vi "Read Results.vi"(8 "error in":errorcluster, 11 "Results Directory":path) -> (0 "error out":errorcluster, 3 "Results":T1[](array[typedef]))   [LabVIEW 2020, in "Peer Review.lvclass"]
uses:
  Peer Review.lvclass
  TypeDefs/File Info.ctl
  TypeDefs/File State.ctl
  TypeDefs/VI Type.ctl
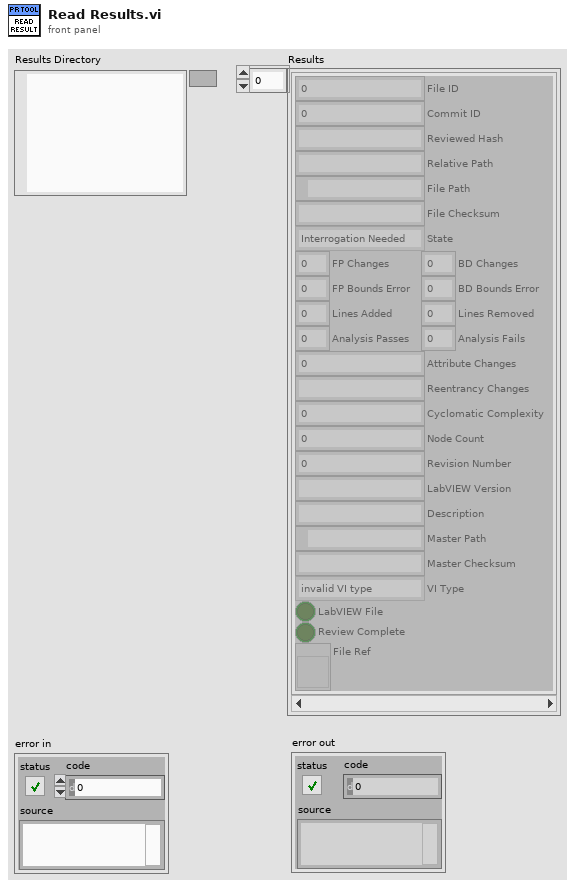
[diagram p1: front panel]
types:
  T1 = typedef "Peer Review.lvclass/File Info.ctl" = cluster{"File ID":i32, "Commit ID":i32, "Reviewed Hash":string, "Relative Path":string, "File Path":path, "File Checksum":string, "State":T2, "FP Changes":i32, "BD Changes":i32, "FP Bounds Error":dbl, "BD Bounds Error":dbl, "Lines Added":i32, "Lines Removed":i32, "Analysis Passes":i32, "Analysis Fails":i32, "Attribute Changes":i32, "Reentrancy Changes":string, "Cyclomatic Complexity":i32, "Node Count":i32, "Revision Number":u32, "LabVIEW Version":string, "Description":string, "Master Path":path, "Master Checksum":string, "VI Type":T3, "LabVIEW File":bool, "Review Complete":bool, "File Ref":refnum<vi>}
  T2 = typedef "Peer Review.lvclass/File State.ctl" = enum16{"Interrogation Needed", "Modified", "Deleted", "Added", "Matches Previous", "No Changes", "Moved"}
  T3 = typedef "Peer Review.lvclass/VI Type.ctl" = enum32{"invalid VI type", "Standard VI", "Control VI", "Global VI", "Polymorphic VI", "Configuration VI", "SubSystem", "Facade VI", "Method VI", "Statechart Diagram VI"}
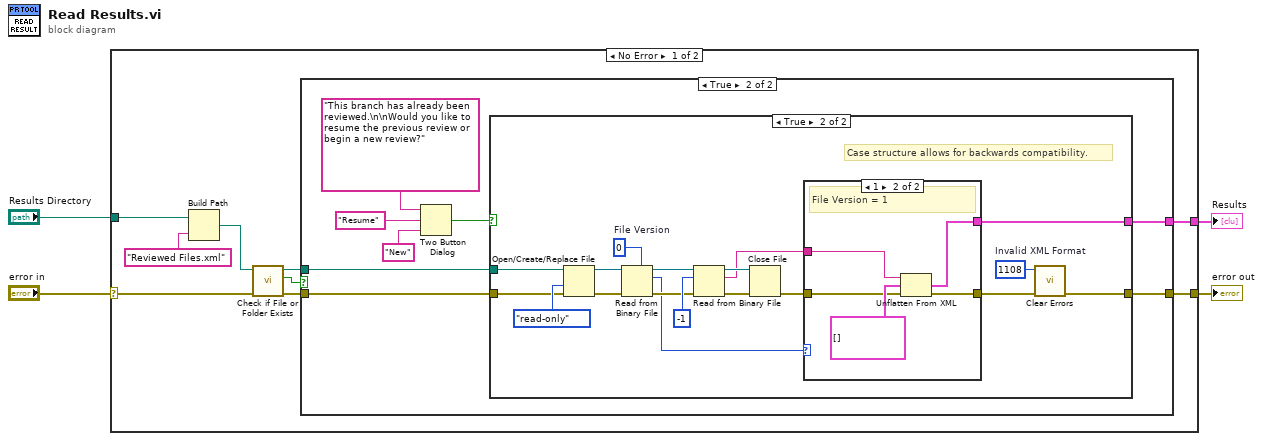
[diagram p0: block diagram]
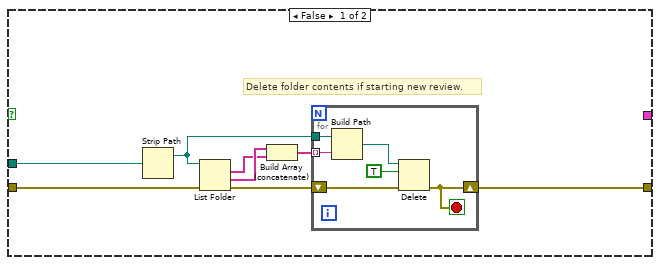
[diagram p3: hidden frame]
diagram:
  n1 = case shown="No Error" "error in" {
    selector: "error in" -> [w11 w61]
    tunnel: "Results Directory" -> [w13 _]
    tunnel: [w6 w61] -> w2
    tunnel: [w5 _] -> w1
    frame No Error {
      n2 = Build Path(base path=w13, name or relative path="Reviewed Files.xml") -> (appended path=w10:path)
      n3 = call <vilib>:"Check if File or Folder Exists.vi"("error in (no error)"=w11, "path"=w10) -> ("error out"=w9:errorcluster, "file or folder exists?"=w8:bool, "dup path"=w7:path)  [unwired: 7 in]
      n4 = case shown="True" w8 {
        tunnel: w9 -> [w14 w18]
        tunnel: w7 -> [_ w22]
        tunnel: [w14 w20] -> w6
        tunnel: [_ w21] -> w5
        frame False {
        }
        frame True {
          n5 = Two Button Dialog(message="This branch has already been reviewed.\n\nWould you like to resume the previous review or begin a new review?", 1:"New" ("F button name (\"Cancel\")"), 2:"Resume" ("T button name (\"OK\")")) -> (T button?=w15:bool)
          n6 = case shown="True" w15 {
            tunnel: w22 -> [w30 w54]
            tunnel: [_ w46] -> w21
            tunnel: [w23 w39] -> w20
            tunnel: w18 -> [w24 w37]
            frame False {
              # "Delete folder contents if starting new review."
              n7 = Strip Path(path=w30) -> (stripped path=w25:path)  [unwired: 1 out]
              n8 = List Folder(path=w25, error in=w24) -> (filenames=w28:string[], folder names=w29:string[], error out=w26:errorcluster)  [unwired: 2 in, 1 out]
              n9 = Build Array (concatenate)(w29, w28) -> (w27:string[])
              n10 = for {
                tunnel: w25 -> [w36]
                tunnel: w27 -> [w35] mode=indexing
                shift-right: [w31] -> w23
                shift-left: w26 -> [w33]
                stop <- w31 stop-if-true
                n11 = Build Path(base path=w36, name or relative path=w35) -> (appended path=w34:path)
                n12 = Delete(path (use dialog)=w34, entire hierarchy (F)=TRUE, error in=w33) -> (error out=w31:errorcluster)  [unwired: 2 in, 2 out]
              }
            }
            frame True {
              w38 = 1108  # Invalid XML Format
              w41 = u32 0  # File Version
              # "Case structure allows for backwards compatibility."
              n13 = Open/Create/Replace File(file path (use dialog)=w54, error in=w37, access (0:read/write)=enum16{"read/write", "read-only", "write-only"}."read-only") -> (refnum out=w45:refnum<file>, error out=w43:errorcluster)  [unwired: 3 in, 1 out]
              n14 = Read from Binary File(5:w41, 8:w43, 11:w45) -> (0:w42:errorcluster, 2:w40:u32, 3:w44:refnum<file>)  [unwired: 3 in, 1 out]
              n15 = Read from Binary File(8:w42, 10:-1 ("count"), 11:w44) -> (0:w50:errorcluster, 2:w48:string, 3:w51:refnum<file>)  [unwired: 3 in, 1 out]
              n16 = Close File(refnum=w51, error in=w50) -> (error out=w49:errorcluster)  [unwired: 1 out]
              n17 = case shown="1" w40 {
                tunnel: w49 -> [w55 w59]
                tunnel: w48 -> [_ w58]
                tunnel: [w55 w57] -> w47
                tunnel: [_ w56] -> w46
                frame Default {
                  # "Invalid file version"
                }
                frame 1 {
                  # "File Version = 1"
                  n18 = Unflatten From XML(xml string=w58, type=T1[] [] ("File Info"), error in (no error)=w59) -> (value=w56:T1[], error out=w57:errorcluster)
                }
              }
              n19 = call <vilib>:"Clear Errors.vi"("error in (no error)"=w47, "specific error code to clear (0: all)"=w38) -> ("error out"=w39:errorcluster)  [unwired: 4 in, 1 out]
            }
          }
        }
      }
    }
    frame Error {
    }
  }
  "error out" <- w2
  "Results" <- w1
